vi "GetWgSwPositions.vi"(4 "error in (no error)":errorcluster) -> (0 "error out":errorcluster, 1 "String_WgSw_Positions":string, 2 "Vout2Ant Position (0=ANT, 1=DL)":i32, 3 "Hout2Ant Position (0=DL, 1=ANT)":i32, 5 "VTxMitch2Ant Position (0=Mitch, 1=Tee)":i32, 6 "HTxMitch2Ant Position (0=Tee, 1=Mitch)":i32, 7 "MainTx2Mitch Position (0=Tee, 1=Mitch)":i32)   [LabVIEW 2009]
doc: "Read all 5 WG switch positions"
panel:
  out "Pol Sw 7223 = 0= SCPI open \"honly\", =1 = SCPI closed \"vonly\"":i32
  out "Pol Sw 7222 = 1 = closed = processor control, = 0 = open = local control":i32
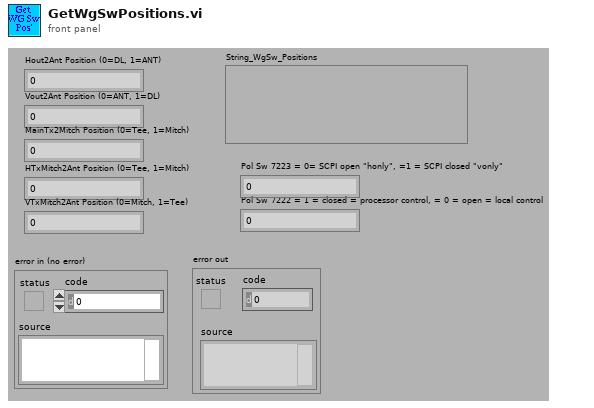
[diagram p1: front panel]
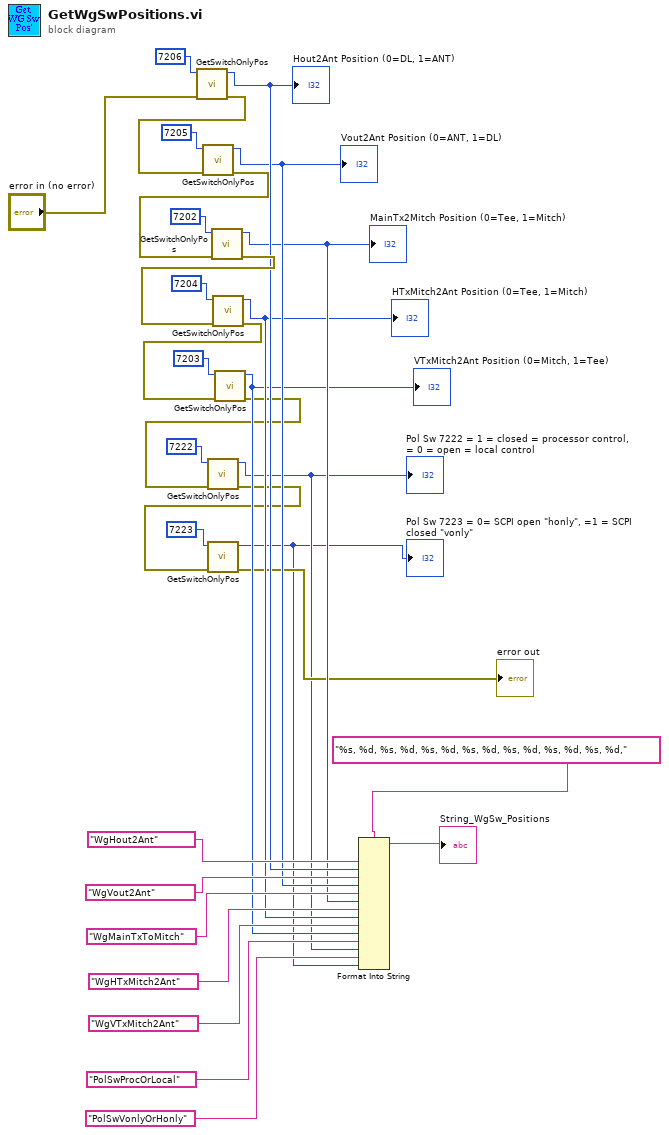
[diagram p0: block diagram]
diagram:
  n1 = call "GetSwitchOnlyPos.vi"("error in (no error)"="error in (no error)", "Circuit ID"=7206) -> ("Error out"=w24:errorcluster, "Position (0=open, 1=closed)"=w14:i32)  [unwired: 4 in]
  "Hout2Ant Position (0=DL, 1=ANT)" <- w14
  n2 = call "GetSwitchOnlyPos.vi"("error in (no error)"=w24, "Circuit ID"=7205) -> ("Error out"=w23:errorcluster, "Position (0=open, 1=closed)"=w13:i32)  [unwired: 4 in]
  "Vout2Ant Position (0=ANT, 1=DL)" <- w13
  n3 = call "GetSwitchOnlyPos.vi"("error in (no error)"=w23, "Circuit ID"=7202) -> ("Error out"=w22:errorcluster, "Position (0=open, 1=closed)"=w12:i32)  [unwired: 4 in]
  "MainTx2Mitch Position (0=Tee, 1=Mitch)" <- w12
  n4 = call "GetSwitchOnlyPos.vi"("error in (no error)"=w22, "Circuit ID"=7204) -> ("Error out"=w20:errorcluster, "Position (0=open, 1=closed)"=w11:i32)  [unwired: 4 in]
  "HTxMitch2Ant Position (0=Tee, 1=Mitch)" <- w11
  n5 = call "GetSwitchOnlyPos.vi"("error in (no error)"=w20, "Circuit ID"=7203) -> ("Error out"=w7:errorcluster, "Position (0=open, 1=closed)"=w10:i32)  [unwired: 4 in]
  "VTxMitch2Ant Position (0=Mitch, 1=Tee)" <- w10
  n6 = call "GetSwitchOnlyPos.vi"("error in (no error)"=w7, "Circuit ID"=7222) -> ("Error out"=w6:errorcluster, "Position (0=open, 1=closed)"=w2:i32)  [unwired: 4 in]
  "Pol Sw 7222 = 1 = closed = processor control, = 0 = open = local control" <- w2
  n7 = call "GetSwitchOnlyPos.vi"("error in (no error)"=w6, "Circuit ID"=7223) -> ("Error out"=→"error out":errorcluster, "Position (0=open, 1=closed)"=w1:i32)  [unwired: 4 in]
  "Pol Sw 7223 = 0= SCPI open \"honly\", =1 = SCPI closed \"vonly\"" <- w1
  n8 = Format Into String(format string="%s, %d, %s, %d, %s, %d, %s, %d, %s, %d, %s, %d, %s, %d,", "WgHout2Ant", w14, "WgVout2Ant", w13, "WgMainTxToMitch", w12, "WgHTxMitch2Ant", w11, "WgVTxMitch2Ant", w10, "PolSwProcOrLocal", w2, "PolSwVonlyOrHonly", w1) -> (resulting string=→"String_WgSw_Positions":string)  [unwired: 2 in, 1 out]
